vi "Car Wash Timer.vi"(7 "Input  State":enum16{"Start Timer", "Check Timer"}(ring), 8 "error in (no error)":errorcluster, 11 "Timer Length":dbl) -> (0 "error out":errorcluster, 2 "Time Elapsed":bool, 3 "Elapsed Time":dbl)   [LabVIEW 2020]
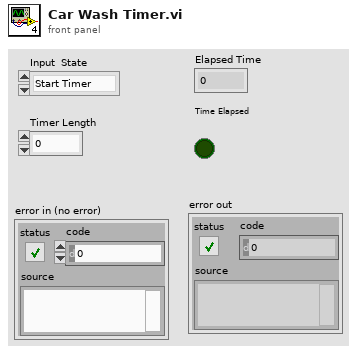
[diagram p1: front panel]
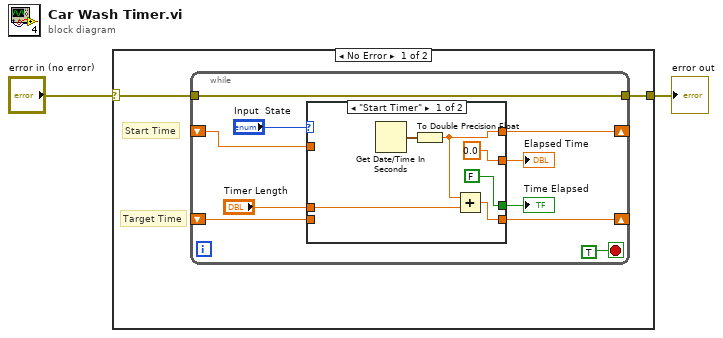
[diagram p0: block diagram]
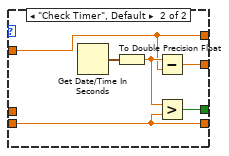
[diagram p2: hidden frame]
diagram:
  n1 = case shown="No Error" "error in (no error)" {
    selector: "error in (no error)" -> [w4 w27]
    tunnel: [w3 w27] -> w1
    frame No Error {
      # "Target Time"
      # "Start Time"
      n2 = while {
        tunnel: w4 -> [w14]
        tunnel: [w14] -> w3
        shift-right: [w10] -> _
        shift-left: _ -> [w8]
        shift-right: [w9] -> _
        shift-left: _ -> [w7]
        stop <- TRUE stop-if-true
        n3 = case shown="\"Start Timer\"" "Input  State" {
          tunnel: "Timer Length" -> [w18 _]
          tunnel: [w19 w22] -> w10
          tunnel: [w17 w21] -> w9
          tunnel: w8 -> [_ w22]
          tunnel: w7 -> [_ w21]
          tunnel: [FALSE w25] -> w6
          tunnel: [0.0 w24] -> w5
          frame "Start Timer" {
            n4 = Get Date/Time In Seconds() -> (seconds since 1Jan1904=w20:timestamp)
            n5 = To Double Precision Float(number=w20) -> (double precision float=w19:dbl)
            n6 = Add(x=w19, y=w18) -> (x+y=w17:dbl)
          }
          frame "Check Timer", Default {
            n7 = Get Date/Time In Seconds() -> (seconds since 1Jan1904=w26:timestamp)
            n8 = To Double Precision Float(number=w26) -> (double precision float=w23:dbl)
            n9 = Subtract(x=w23, y=w22) -> (x-y=w24:dbl)
            n10 = Greater?(x=w23, y=w21) -> (0:w25:bool)
          }
        }
        "Elapsed Time" <- w5
        "Time Elapsed" <- w6
      }
    }
    frame Error {
    }
  }
  "error out" <- w1
